vi "valve - Copy.vi"(0 "X(State)":T2={"X2(MenuCmdSource)"=1, "X3(MenuSetSate)"=enum."on", "X4(AutoSetState)"=enum."on", "X5(DistSetSate)"=enum."on"}, 1 "XB01":bool, 2 "XB02":bool, 3 "XB24":bool, 4 "Valve parameters table":u32[](array[numeric])=[1000, 10000, 300, 300, 3000, 5000, 5000], 6 "ALRL2":bool, 8 "ALRL1":bool) -> (10 "reset out":bool, 12 "This VI":refnum<vi>, 14 "Z":T1, 17 "YB02 (no stop)":bool, 18 "YB01 (on)":bool, 19 "ALR_ON":bool[](array[boolean]))   [LabVIEW 2015, in "Userlib.lvlib"]
uses:
  Userlib.lvlib
  Counter/Generator.vi
panel:
  in  "on":bool
  in  "auto":bool
  in  "reset":bool
  out "alarm ind":u16(ring)
  out "Z1 ind":u8(ring)
  out "Z3 ind":u16(ring)
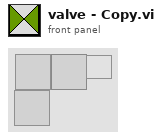
[diagram p1: front panel]
types:
  T1 = cluster{"Z1(CmdSource)":enum8{"local disabled", "local hand", "hand", "auto", "dist"}, "Z3(State)":enum8{"alarm", "disabled", "not ready", "stop ready", "reserv", "switched off", "switched on", "check", "on min", "decrease speed", "on", "increase speed", "on max"}, "Z5":u8}
  T2 = cluster{"X2(MenuCmdSource)":u8, "X3(MenuSetSate)":enum8{"alarm", "disabled", "not ready", "stop ready", "reserv", "switched off", "switched on", "check", "on min", "decrease speed", "on", "increase speed", "on max"}, "X4(AutoSetState)":enum8{"alarm", "disabled", "not ready", "stop ready", "reserv", "switched off", "switched on", "check", "on min", "decrease speed", "on", "increase speed", "on max"}, "X5(DistSetSate)":enum8{"alarm", "disabled", "not ready", "stop ready", "reserv", "switched off", "switched on", "check", "on min", "decrease speed", "on", "increase speed", "on max"}}
  T3 = enum8{"alarm", "disabled", "not ready", "stop ready", "reserv", "switched off", "switched on", "check", "on min", "decrease speed", "on", "increase speed", "on max"}
  T4 = enum8{"local disabled", "local hand", "hand", "auto", "dist"}
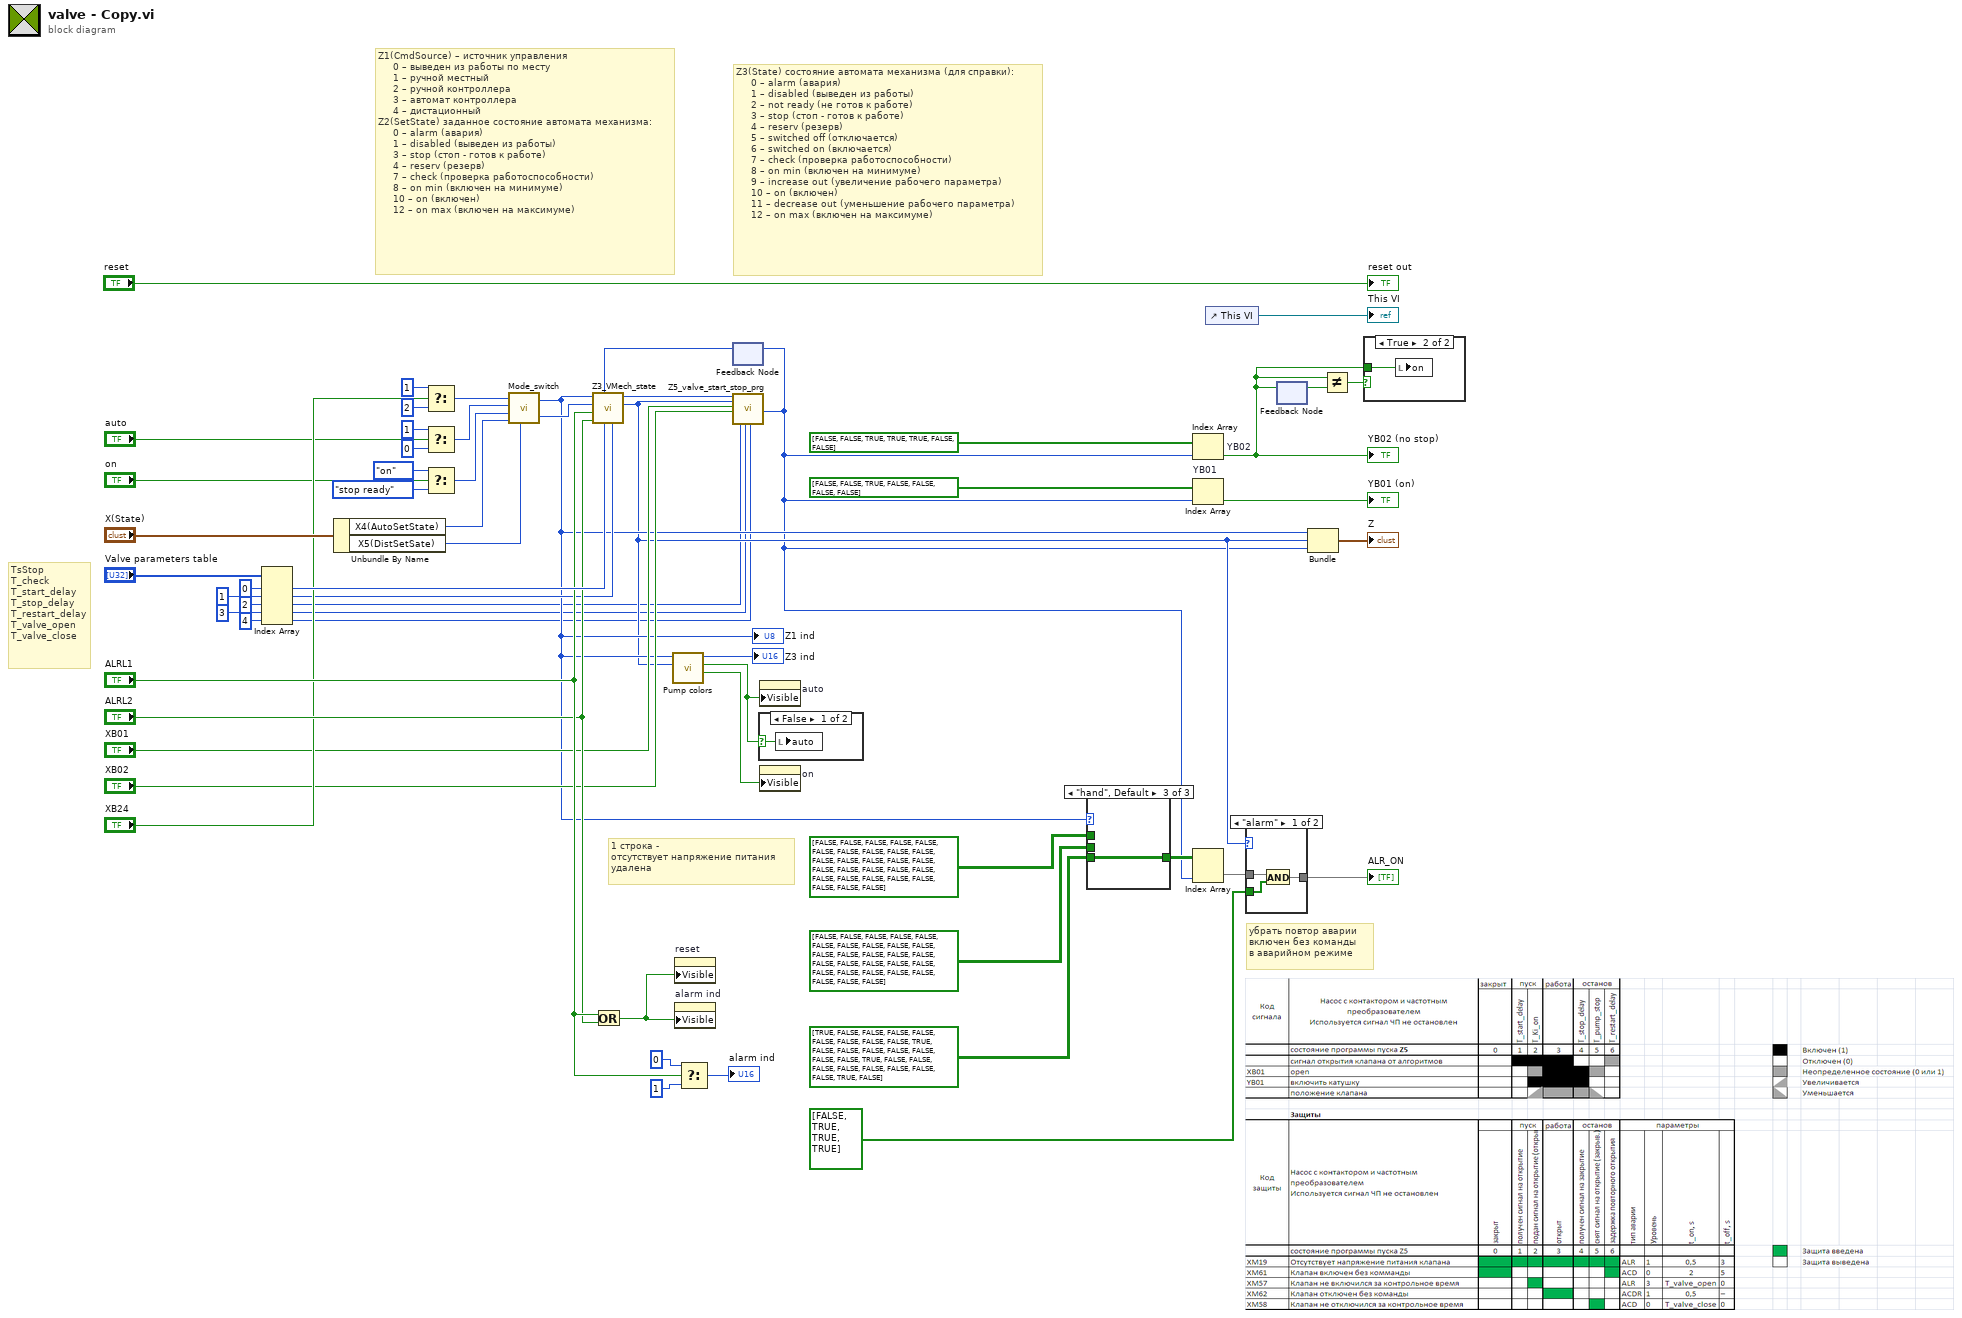
[diagram p0: block diagram]
diagram:
  # "1 строка - \nотсутствует напряжение питания\nудалена"
  # "убрать повтор аварии\nвключен без команды\nв аварийном режиме"
  # "TsStop\nT_check\nT_start_delay\nT_stop_delay\nT_restart_delay\nT_valve_open\nT_valve_close"
  # "Z1(CmdSource) – источник управления\n     0 – выведен из работы по месту\n     1 – ручной местный\n     2 – ручной контроллера\n     3 – автомат контроллера\n     4 – дистационный\nZ2(SetState) заданное состояние автомата механизма:\n     0 – alarm (авария)\n     1 – disabled (выведен из работы)\n     3 – stop (стоп - готов к работе)\n     4 – reserv (резерв)\n     7 – check (проверка работоспособности)\n     8 – on min (включен на минимуме)\n     10 – on (включен)\n     12 – on max (включен на максимуме)"
  # "Z3(State) состояние автомата механизма (для справки):\n     0 – alarm (авария)\n     1 – disabled (выведен из работы)\n     2 – not ready (не готов к работе)\n     3 – stop (стоп - готов к работе)\n     4 – reserv (резерв)\n     5 – switched off (отключается)\n     6 – switched on (включается)\n     7 – check (проверка работоспособности)\n     8 – on min (включен на минимуме)\n     9 – increase out (увеличение рабочего параметра)\n     10 – on (включен)\n     11 – decrease out (уменьшение рабочего параметра)\n     12 – on max (включен на максимуме)"
  n1 = Index Array(array="Valve parameters table", index #1=0 ("index"), index #2=1 ("index"), index #3=2 ("index"), index #4=3 ("index"), index #5=4 ("index")) -> (element #1=w40:u32, element #2=w8:u32, element #3=w1:u32, element #4=w2:u32, element #5=w3:u32)
  n2 = Unbundle By Name("X(State)") -> ("X4(AutoSetState)"=w32:T3, "X5(DistSetSate)"=w31:T3)
  n3 = Select(t=u32 1, s="XB24", f=u32 2) -> (s? t:f=w41:u32)
  n4 = Select(t=u32 1, s="auto", f=u32 0) -> (s? t:f=w20:u32)
  n5 = Select(t=T3."on" ("X3(MenuSetSate)"), s="on", f=T3."stop ready" ("X3(MenuSetSate)")) -> (s? t:f=w19:T3)
  n6 = call "Mode_switch.vi"("X1(HSwitch)"=w41, "X2(MenuCmdSource)"=w20, "X3(MenuSetSate)"=w19, "X4(AutoSetState)"=w32, "X5(DistSetSate)"=w31) -> ("Z1(CmdSource)"=w6:T4, "Z2(SetState)"=w42:T3)
  "Z1 ind" <- w6
  n7 = Or(x="ALRL1", y="ALRL2") -> (x .or. y?=w51:bool)
  n8 = property on="reset" class="Bool (strict)"("Visible"=w51) -> ()  [unwired: 2 in, 2 out]
  n9 = property on="alarm ind" class="Ring (strict)"("Visible"=w51) -> ()  [unwired: 2 in, 2 out]
  n10 = Select(t=u16 0 ("alarm ind"), s="ALRL1", f=u16 1 ("alarm ind")) -> (s? t:f=→"alarm ind":u16)
  n11 = feedback #1() -> (w43:u8)  [unwired: 1 in]
  n12 = call "Z3_VMech_state.vi"("t_check"=w8, "TsStop"=w40, "Z5"=w43, "Alarm_L2"="ALRL2", "Alarm_L1"="ALRL1", "Z2(SetState)"=w42, "Z1(CmdSource)"=w6) -> ("Z3(State)"=w5:T3, "Z1_Out"=w59:T4)  [unwired: 2 in, 1 out]
  n13 = call "Pump colors.vi"("Z3(Sate)"=w5, "Z1(CmdSource)"=w6) -> ("on visible"=w18:bool, "auto visible"=w13:bool, "N ring"=→"Z3 ind":u16)  [unwired: 6 in, 1 out]
  n14 = call "Z5_valve_start_stop_prg.vi"("Z1(CmdSource)"=w59, "Z3(State)"=w5, "open"="XB01", "close"="XB02", "T_start_delay"=w1, "T_stop_delay"=w2, "T_restart_delay"=w3) -> ("Z5"=w4:u8)  [unwired: 8 in, 4 out]
  n15 = feedback-in #1(w4) -> ()
  n16 = case shown="False" w13 {
    selector: w13 -> [w60 _]
    frame False {
      n17 = local write "auto"(w60) -> ()
    }
    frame True {
    }
  }
  n18 = property on="auto" class="Bool (strict)"("Visible"=w13) -> ()  [unwired: 2 in, 2 out]
  n19 = property on="on" class="Bool (strict)"("Visible"=w18) -> ()  [unwired: 2 in, 2 out]
  n20 = case shown="\"hand\", Default" w6 {
    tunnel: bool[][] [[FALSE, FALSE, FALSE, FALSE, FALSE, FALSE, FALSE], [FALSE, FALSE, FALSE, FALSE, FALSE, FALSE, FALSE], [FALSE, FALSE, FALSE, FALSE, FALSE, FALSE, FALSE], [FALSE, FALSE, FALSE, FALSE, FALSE, FALSE, FALSE]] -> [w61 _ _]
    tunnel: bool[][] [[FALSE, FALSE, FALSE, FALSE, FALSE, FALSE, FALSE], [FALSE, FALSE, FALSE, FALSE, FALSE, FALSE, FALSE], [FALSE, FALSE, FALSE, FALSE, FALSE, FALSE, FALSE], [FALSE, FALSE, FALSE, FALSE, FALSE, FALSE, FALSE]] -> [_ w62 _]
    tunnel: bool[][] [[TRUE, FALSE, FALSE, FALSE, FALSE, FALSE, FALSE], [FALSE, FALSE, TRUE, FALSE, FALSE, FALSE, FALSE], [FALSE, FALSE, FALSE, TRUE, FALSE, FALSE, FALSE], [FALSE, FALSE, FALSE, FALSE, FALSE, TRUE, FALSE]] -> [_ _ w63]
    tunnel: [w61 w62 w63] -> w34
    frame "local disabled" {
    }
    frame "local hand" {
    }
    frame "hand", Default {
    }
  }
  n21 = Index Array "YB02"(array=bool[] [FALSE, FALSE, TRUE, TRUE, TRUE, FALSE, FALSE], index=w4) -> (element=w15:bool)
  "YB02 (no stop)" <- w15
  n22 = Index Array "YB01"(array=bool[] [FALSE, FALSE, TRUE, FALSE, FALSE, FALSE, FALSE], index=w4) -> (element=→"YB01 (on)":bool)
  n23 = Index Array(array=w34, index (col)=w4) -> (element=w28:bool[])  [unwired: 1 in]
  n24 = control-ref of="This VI"() -> (→"This VI":refnum<vi>)
  n25 = case shown="\"alarm\"" w5 {
    tunnel: bool[] [FALSE, TRUE, TRUE, TRUE] -> [w65 _]
    tunnel: w28 -> [w66 w67]
    tunnel: [w64 w67] -> w27
    frame "alarm" {
      n26 = And(x=w66, y=w65) -> (x .and. y?=w64:bool[])
    }
    frame "disabled", Default {
    }
  }
  "ALR_ON" <- w27
  n27 = feedback #2() -> (w17:bool)  [unwired: 1 in]
  n28 = feedback-in #2(w15) -> ()
  n29 = Bundle("Z1(CmdSource)"=w6, "Z3(State)"=w5, "Z5"=w4) -> (→"Z":T1)  [unwired: 1 in]
  n30 = Not Equal?(x=w15, y=w17) -> (x != y?=w16:bool)
  n31 = case shown="True" w16 {
    tunnel: w15 -> [_ w68]
    frame False {
    }
    frame True {
      n32 = local write "on"(w68) -> ()
    }
  }
  "reset out" <- "reset"
